vi "HP-S-test.vi"() -> ()   [LabVIEW 2020, in "HP-S-Serial.lvclass"]
uses:
  HP-S-Serial.lvclass
  HP-S-session.ctl
  HP-S-data.ctl
  HP-S-settings.ctl
  HP-S-baudrate.ctl
  HP-S-Serial.lvclass/HP-S-Serial.ctl
  93c78fef-5040-4ae5-938b-63389a54b8ad.vi
panel:
  out "error out":errorcluster
  out "send":T1 format="%x"
  out "req":T1=[16, 13] format="%x"
  out "req 2":T1 format="%x"
  out "req out":T1 format="%x"
  out "session":T2 {"last get" format="%x"; "last set" format="%x"}
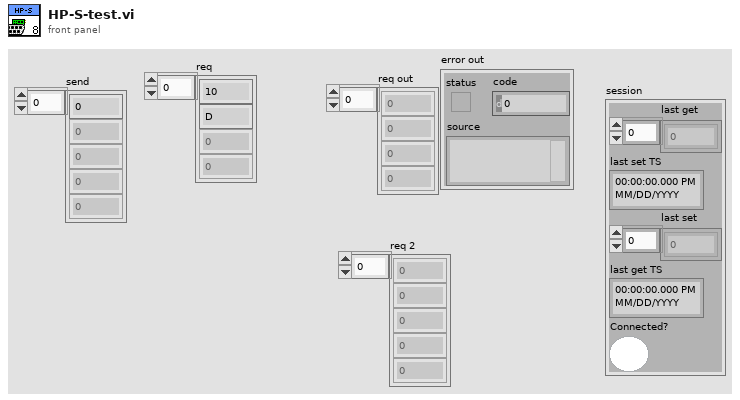
[diagram p1: front panel]
types:
  T1 = typedef "HP-S-Serial.lvclass/HP-S-data.ctl" = u8[]
  T2 = typedef "HP-S-Serial.lvclass/HP-S-session.ctl" = cluster{"last get":T1, "last set TS":timestamp, "last set":T1, "last get TS":timestamp, "Connected?":bool}
  T3 = typedef "HP-S-Serial.lvclass/HP-S-settings.ctl" = cluster{"VISA resource name":refnum<visa-resource-name>, "baud rate (9600)":T4, "timeout (10sec)":u32, "termination char\n(0xA = '\\n' = LF) ":u8, "Enable Termination\nChar (T)":bool, "data bits (8)":u16, "parity (0:none)":enum16{"None", "Odd", "Even", "Mark", "Space"}}
  T4 = typedef "HP-S-Serial.lvclass/HP-S-baudrate.ctl" = u32
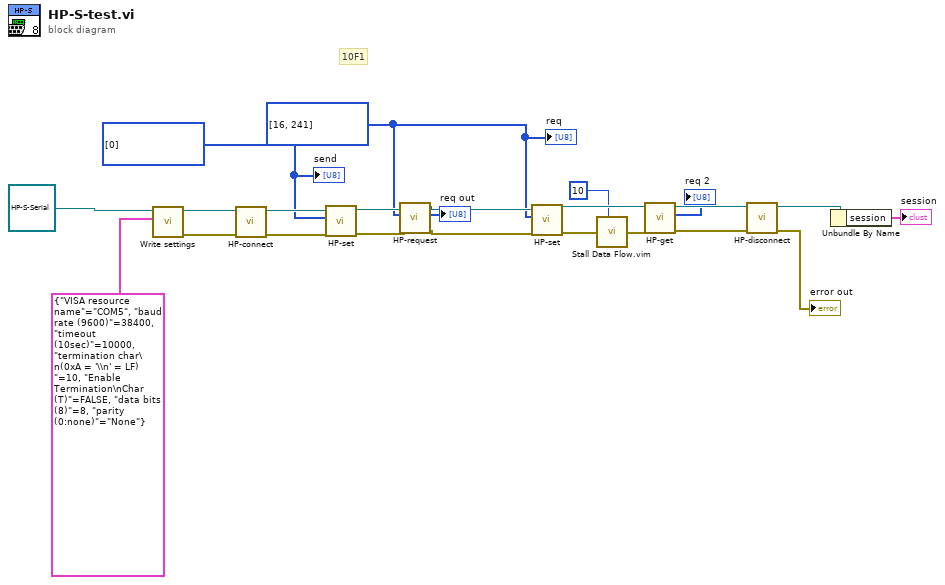
[diagram p0: block diagram]
diagram:
  w4 = T1 [16, 241] ("8bit array")
  w5 = T1 [0] ("8bit array")
  # "10F1"
  n1 = call-dynamic "Write settings.vi"("settings"=T3 {"VISA resource name"="COM5", "baud rate (9600)"=38400, "timeout (10sec)"=10000, "termination char\n(0xA = '\\n' = LF) "=10, "Enable Termination\nChar (T)"=FALSE, "data bits (8)"=8, "parity (0:none)"=enum."None"}, "HP-S-Serial in"=refnum<class "HP-S-Serial.lvclass"> refnum) -> ("error out"=w22:errorcluster, "HP-S-Serial out"=w23:refnum<class "HP-S-Serial.lvclass">)  [unwired: 8 in]
  n2 = call-dynamic "HP-connect.vi"("error in (no error)"=w22, "HP-S-Serial in"=w23) -> ("error out"=w20:errorcluster, "HP-S-Serial out"=w21:refnum<class "HP-S-Serial.lvclass">)  [unwired: 8 in]
  n3 = call-dynamic "HP-set.vi"("error in (no error)"=w20, "write buffer"=w5, "HP-S-Serial in"=w21) -> ("error out"=w18:errorcluster, "HP-S-Serial out"=w19:refnum<class "HP-S-Serial.lvclass">)  [unwired: 7 in]
  n4 = call-dynamic "HP-request.vi"("error in (no error)"=w18, "write buffer"=w4, "HP-S-Serial in"=w19) -> ("error out"=w10:errorcluster, "read buffer"=→"req out":T1, "HP-S-Serial out"=w11:refnum<class "HP-S-Serial.lvclass">)  [unwired: 6 in]
  n5 = call-dynamic "HP-set.vi"("error in (no error)"=w10, "write buffer"=w4, "HP-S-Serial in"=w11) -> ("error out"=w9:errorcluster, "HP-S-Serial out"=w8:refnum<class "HP-S-Serial.lvclass">)  [unwired: 7 in]
  n6 = call "Stall Data Flow.vim"("value in"=w9, "milliseconds to wait"=u32 10) -> ("value out"=w2:errorcluster)  [unwired: 1 out]
  n7 = call-dynamic "HP-get.vi"("error in (no error)"=w2, "HP-S-Serial in"=w8) -> ("error out"=w16:errorcluster, "read buffer"=→"req 2":T1, "HP-S-Serial out"=w17:refnum<class "HP-S-Serial.lvclass">)  [unwired: 7 in]
  n8 = call-dynamic "HP-disconnect.vi"("error in (no error)"=w16, "HP-S-Serial in"=w17) -> ("error out"=→"error out":errorcluster, "HP-S-Serial out"=w13:refnum<class "HP-S-Serial.lvclass">)  [unwired: 8 in]
  n9 = Unbundle By Name(w13) -> ("session"=→"session":T2)
  "req" <- w4
  "send" <- w5
